vi "Turn On.vi"(8 "error in (no error)":errorcluster, 11 "Lamp in":refnum<class "Lamp.lvclass">) -> (0 "error out":errorcluster, 3 "Lamp out":refnum<class "Lamp.lvclass">)   [LabVIEW 2018, in "Lamp.lvclass"]
uses:
  Lamp.lvclass
  Switchable Device/Switchable Device.lvclass
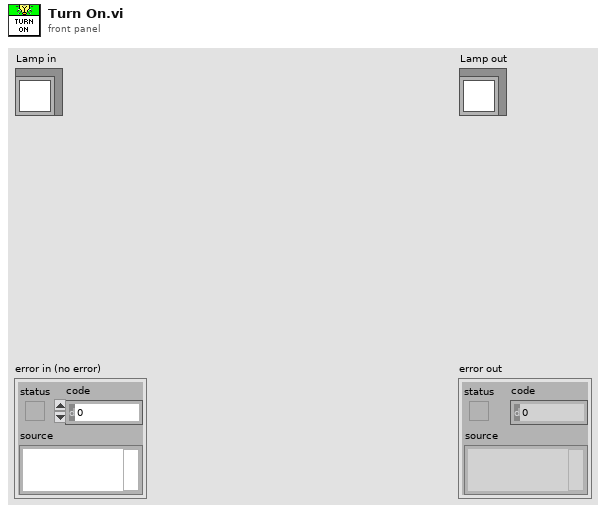
[diagram p1: front panel]
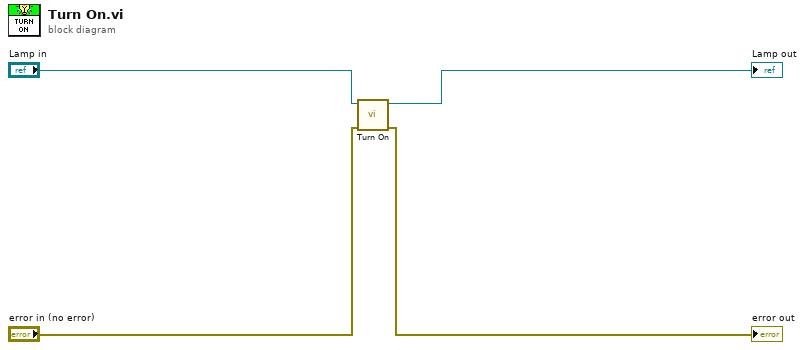
[diagram p0: block diagram]
diagram:
  n1 = call-parent "Turn On.vi"("error in (no error)"="error in (no error)", "Switchable Device in"="Lamp in") -> ("error out"=→"error out":errorcluster, "Switchable Device out"=→"Lamp out":refnum<class "Lamp.lvclass">)  [unwired: 8 in]
